vi "ke2000 Configure Route Multiple.vi"(0 "VISA resource name":refnum<visa-resource-name>, 1 "Operation (0: Open All)":u16(ring) items=["Open All", "Open", "Close"], 2 "Channels (Empty)":i32[](array[numeric]), 5 "error in (no error)":errorcluster) -> (14 "VISA resource name out":refnum<visa-resource-name>, 19 "error out":errorcluster)   [LabVIEW 2010]
doc: "This VI controls the switch functionality of an internal or external scanner card. It can be used to open or close one or more channels.\n\nNote:\nThis is a polymorphic VI. You can wire a single channel number or an array of channel numbers to configure multiple channels at once."
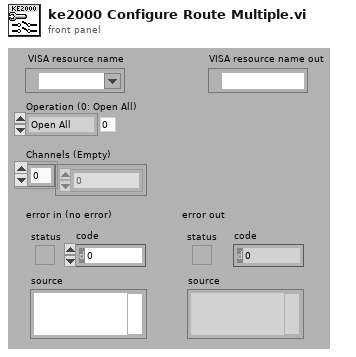
[diagram p1: front panel]
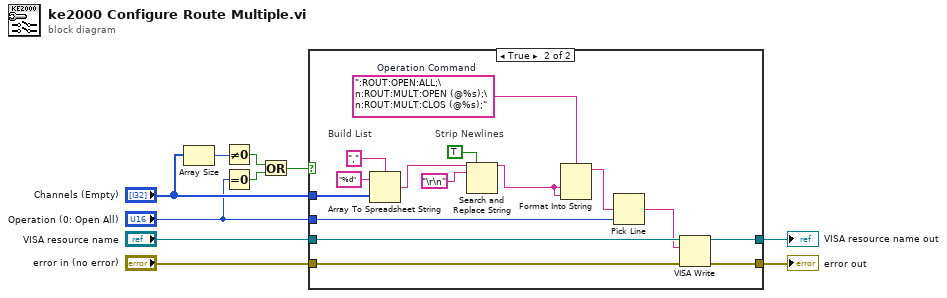
[diagram p0: block diagram]
diagram:
  n1 = Array Size(array="Channels (Empty)") -> (size(s)=w5:i32)
  n2 = Not Equal To 0?(x=w5) -> (x != 0?=w3:bool)
  n3 = Equal To 0?(x="Operation (0: Open All)") -> (x = 0?=w2:bool)
  n4 = Or(x=w3, y=w2) -> (x .or. y?=w1:bool)
  n5 = case shown="True" w1 {
    tunnel: "VISA resource name" -> [w12 w27]
    tunnel: "error in (no error)" -> [w11 w26]
    tunnel: [w12 w25] -> w8
    tunnel: [w11 w24] -> w7
    tunnel: "Operation (0: Open All)" -> [_ w21]
    tunnel: "Channels (Empty)" -> [_ w17]
    frame False {
    }
    frame True {
      w23 = ":ROUT:OPEN:ALL;\n:ROUT:MULT:OPEN (@%s);\n:ROUT:MULT:CLOS (@%s);"  # Operation Command
      # "Strip Newlines"
      # "Build List"
      n6 = Array To Spreadsheet String(delimiter (Tab)=",", array=w17, 3:"%d" ("format string")) -> (spreadsheet string=w15:string)
      n7 = Search and Replace String(replace all?=TRUE ("replace all? (F)"), input string=w15, search string="\r\n") -> (result string=w14:string)  [unwired: 5 in, 3 out]
      n8 = Format Into String(format string=w23, w14, w14) -> (resulting string=w22:string)  [unwired: 2 in, 1 out]
      n9 = Pick Line(multi-line string=w22, line index=w21) -> (output string=w20:string)  [unwired: 1 in]
      n10 = VISA Write(VISA resource name=w27, write buffer=w20, error in (no error)=w26) -> (VISA resource name out=w25:refnum<visa-resource-name>, error out=w24:errorcluster)  [unwired: 1 out]
    }
  }
  "error out" <- w7
  "VISA resource name out" <- w8
